vi "Get Unbundler Input Terminal.vi"(8 "error in (no error)":errorcluster, 11 "Unbundler in":refnum<vi>) -> (0 "error out":errorcluster, 2 "Unbundle Input Term Refnum":refnum<vi>, 3 "Unbundler out":refnum<vi>)   [LabVIEW 2019, in "gRPC Template Creation Utility.lvlib"]
uses:
  gRPC Template Creation Utility.lvlib
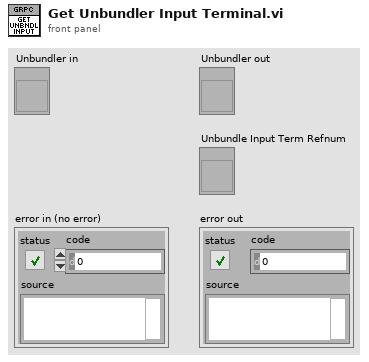
[diagram p1: front panel]
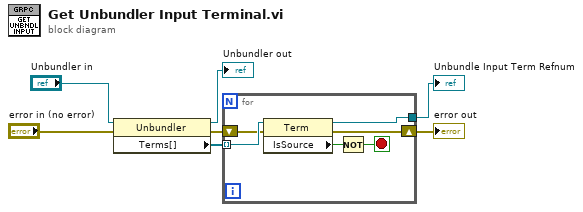
[diagram p0: block diagram]
diagram:
  n1 = property class="Unbundler"(reference="Unbundler in", error in="error in (no error)") -> (reference out=→"Unbundler out":refnum<vi>, error out=w5:errorcluster, "Terms[]"=w3:refnum<vi>[])
  n2 = for {
    tunnel: w3 -> [w13] mode=indexing
    shift-right: [w11] -> w7
    shift-left: w5 -> [w9]
    tunnel: [w12] -> w6
    stop <- w8 stop-if-true
    n3 = property class="Term"(reference=w13, error in=w9) -> (reference out=w12:refnum<vi>, error out=w11:errorcluster, "IsSource"=w10:bool)
    n4 = Not(x=w10) -> (.not. x?=w8:bool)
  }
  "error out" <- w7
  "Unbundle Input Term Refnum" <- w6
